vi "InspectTellCleanup.vi"(6 "Error":errorcluster, 7 "Actor":refnum<class "Actor.lvclass">, 10 "PreInspectTellError":errorcluster, 11 "Message":refnum<class "Msg.lvclass">) -> (4 "Error":errorcluster, 5 "Actor":refnum<class "Actor.lvclass">)   [LabVIEW 2020, in "_Template.lvlib" / "{{Actor}}.lvlib" / "Actor.lvclass"]
uses:
  jettl/jettl/Msg/Msg.lvclass
  Actor.lvclass
  Actor.lvclass/Actor.ctl
  jettl/jettl/Actor/Actor.lvclass
panel:
  # "This front panel should not be manipulated."
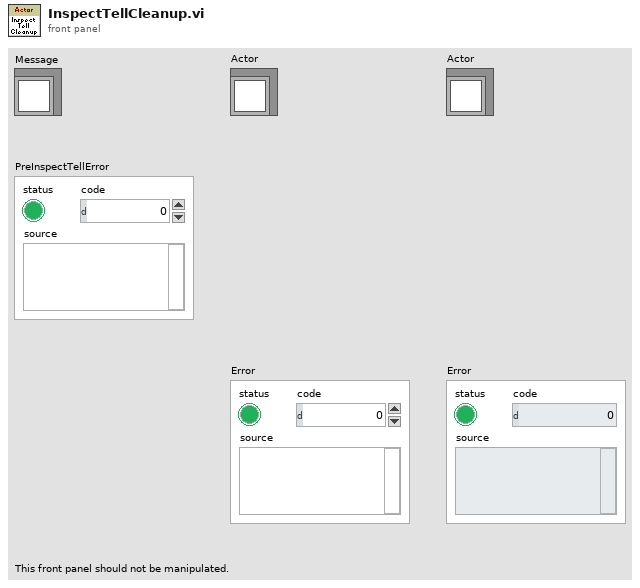
[diagram p1: front panel]
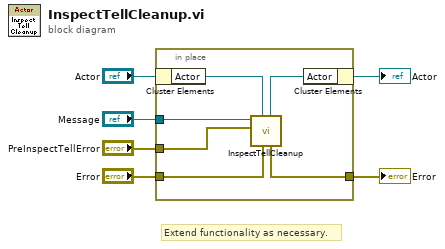
[diagram p0: block diagram]
diagram:
  # "Extend functionality as necessary."
  n1 = in-place {
    in-place-border: "Message" -> [w10]
    in-place-border: "PreInspectTellError" -> [w9]
    in-place-border: "Error" -> [w8]
    in-place-border: [w7] -> w1
    n2 = in-place-cluster #1("Actor") -> ("Actor"=w12:refnum<class "Actor.lvclass">)
    n3 = call-dynamic "InspectTellCleanup.vi"("Error"=w8, "Actor"=w12, "PreInspectTellError"=w9, "Message"=w10) -> ("Error"=w7:errorcluster, "Actor"=w11:refnum<class "Actor.lvclass">)  [unwired: 6 in]
    n4 = in-place-cluster #1("Actor"=w11) -> (→"Actor":refnum<class "Actor.lvclass">)
  }
  "Error" <- w1
